vi "Configure Safety Settings.vi"(6 "Safety Limits":T2={"Temperature Limit (C)"=80, "Low Voltage Limit (V)"=5.0, "High Voltage Limit (V)"=25.0, "Maximum Torque%"=100.0}, 8 "error in (no error)":errorcluster, 9 "Alarm Settings":cluster{"LED Alarm":T1, "Shutdown Alarm":T1}={"LED Alarm"={"Input Voltage"=TRUE, "Angle Limit"=FALSE, "Overheating "=TRUE, "Range"=FALSE, "Checksum"=FALSE, "Overload"=FALSE, "Instruction"=FALSE}, "Shutdown Alarm"={"Input Voltage"=TRUE, "Angle Limit"=FALSE, "Overheating "=TRUE, "Range"=FALSE, "Checksum"=FALSE, "Overload"=FALSE, "Instruction"=FALSE}}, 10 "Motor ID (0)":u8, 11 "Dynamixel Motor VISA in":refnum<class "Dynamixel Motor VISA.lvclass">) -> (0 "error out":errorcluster, 3 "Dynamixel Motor VISA out":refnum<class "Dynamixel Motor VISA.lvclass">)   [LabVIEW 2016, in "Dynamixel Motor VISA.lvclass"]
doc: "Sets limits for the temperature, voltage, and torque for the motor as well as the action to take for status errors for: temperature, overload, angle limit, checksum, etc."
uses:
  <instrlib>/Dynamixel Motor/HAIOL/VISA/Dynamixel Motor VISA.lvclass
  <instrlib>/Dynamixel Motor/Public/Motor Operation/Low Level/Alarm Setting.ctl
  <instrlib>/Dynamixel Motor/HAIOL/VISA/Dynamixel Motor VISA.lvclass/Dynamixel Motor VISA.ctl
  <instrlib>/Dynamixel Motor/Dynamixel Motor.lvlib
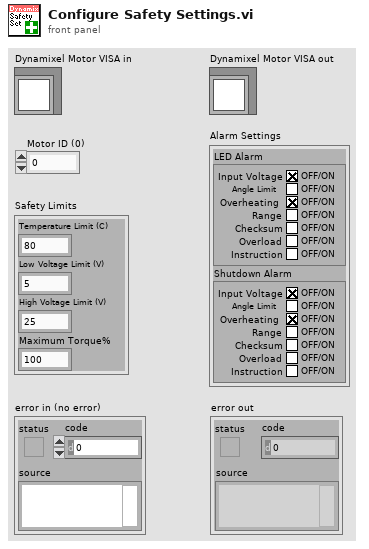
[diagram p1: front panel]
types:
  T1 = typedef "Dynamixel Motor.lvlib/Alarm Setting.ctl" = cluster{"Input Voltage":bool, "Angle Limit":bool, "Overheating ":bool, "Range":bool, "Checksum":bool, "Overload":bool, "Instruction":bool}
  T2 = cluster{"Temperature Limit (C)":u8, "Low Voltage Limit (V)":dbl, "High Voltage Limit (V)":dbl, "Maximum Torque%":dbl}
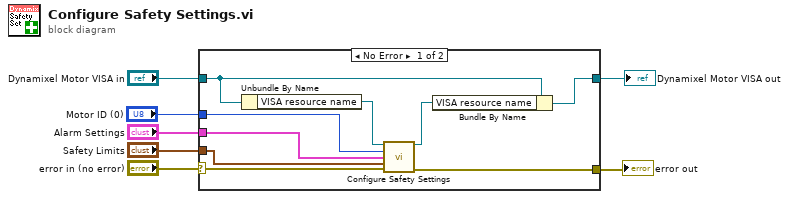
[diagram p0: block diagram]
diagram:
  n1 = case shown="No Error" "error in (no error)" {
    selector: "error in (no error)" -> [w16 w17]
    tunnel: "Dynamixel Motor VISA in" -> [w9 w18]
    tunnel: "Motor ID (0)" -> [w14 _]
    tunnel: "Alarm Settings" -> [w13 _]
    tunnel: "Safety Limits" -> [w12 _]
    tunnel: [w11 w17] -> w2
    tunnel: [w8 w18] -> w1
    frame No Error {
      n2 = Unbundle By Name(w9) -> ("VISA resource name"=w15:refnum<visa-resource-name>)
      n3 = call <instrlib>:"Configure Safety Settings.vi"("VISA resource name"=w15, "Motor ID (0)"=w14, "Alarm Settings"=w13, "Safety Limits"=w12, "error in (no error)"=w16) -> ("VISA resource name out"=w10:refnum<visa-resource-name>, "error out"=w11:errorcluster)  [unwired: 9 in]
      n4 = Bundle By Name(cluster=w9, "VISA resource name"=w10) -> (w8:refnum<class "Dynamixel Motor VISA.lvclass">)
    }
    frame Error {
    }
  }
  "error out" <- w2
  "Dynamixel Motor VISA out" <- w1
